vi "Set Facility Level.vi"(8 "error in (no error)":errorcluster, 10 "Level":T1, 11 "Facility":T2) -> (0 "error out":errorcluster)   [LabVIEW 2017, in "Log.lvclass"]
uses:
  Log.lvclass
  Log_Facilities.ctl
  Log_Level.ctl
  Log_Facility.ctl
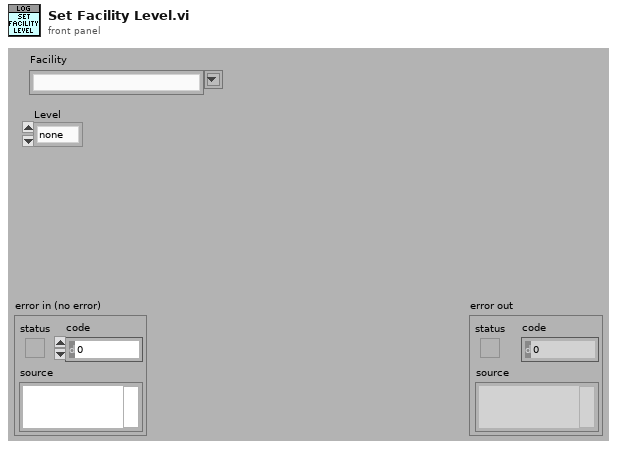
[diagram p1: front panel]
types:
  T1 = typedef "Log.lvclass/Log_Level.ctl" = enum16{"none", "info", "trace", "warn", "error", "fatal"}
  T2 = typedef "Log.lvclass/Log_Facilities.ctl" = string
  T3 = typedef "Log.lvclass/Log_Facility.ctl" = cluster{"Path":path, "Ref":refnum<file>, "Level":T1}
  T4 = typedef "Log.lvclass/ObjectAttributes.ctl" = cluster{"Level":T1, "Facilities":variant, "Event":refnum<user-event>}
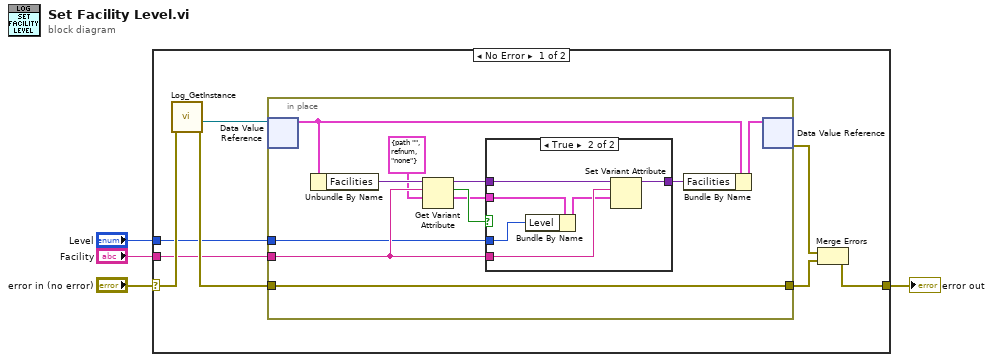
[diagram p0: block diagram]
diagram:
  n1 = case shown="No Error" "error in (no error)" {
    selector: "error in (no error)" -> [w11 w31]
    tunnel: [w5 w31] -> w3
    tunnel: "Facility" -> [w7 _]
    tunnel: "Level" -> [w6 _]
    frame No Error {
      n2 = call "Log_GetInstance.vi"("error in (no error)"=w11) -> ("error out"=w9:errorcluster, "DVRRefOut"=w10:refnum<data-value>)  [unwired: 6 in, 3 out]
      n3 = in-place {
        in-place-border: w9 -> [w22]
        in-place-border: [w22] -> w8
        in-place-border: w7 -> [w17]
        in-place-border: w6 -> [w13]
        n4 = in-place-dvr #1(w10) -> (w20:T4)  [unwired: 1 out]
        n5 = Unbundle By Name(w20) -> ("Facilities"=w21:variant)
        n6 = Get Variant Attribute(Variant=w21, name=w17, default value (empty Variant)=T3 {"Path"=path "", "Ref"=refnum, "Level"=enum."none"} ("Cluster")) -> (duplicate Variant=w19:variant, found=w16:bool, value=w14:T3)  [unwired: 1 in, 1 out]
        n7 = case shown="True" w16 {
          tunnel: w19 -> [w24 w30]
          tunnel: [w24 w29] -> w18
          tunnel: w17 -> [_ w28]
          tunnel: w14 -> [_ w27]
          tunnel: w13 -> [_ w25]
          frame False {
          }
          frame True {
            n8 = Bundle By Name(cluster=w27, "Level"=w25) -> (w26:T3)
            n9 = Set Variant Attribute(Variant=w30, name=w28, value=w26) -> (Variant out=w29:variant)  [unwired: 1 in, 2 out]
          }
        }
        n10 = Bundle By Name(cluster=w20, "Facilities"=w18) -> (w23:T4)
        n11 = in-place-dvr #1(w23) -> (w12:errorcluster)  [unwired: 1 out]
      }
      n12 = Merge Errors(w12, w8) -> (w5:errorcluster)
    }
    frame Error {
    }
  }
  "error out" <- w3
